vi "CalcTheta.vi"() -> (3 "ThetaValues":dbl[](array[numeric]))   [LabVIEW 2018]
panel:
  # "Front of bot"
  # "L"
  # "W"
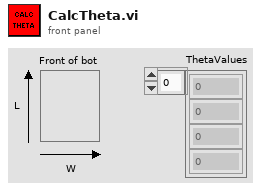
[diagram p1: front panel]
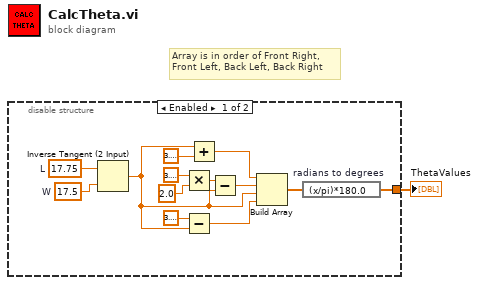
[diagram p0: block diagram]
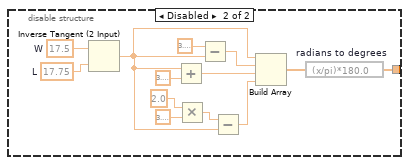
[diagram p2: hidden frame]
diagram:
  # "Array is in order of Front Right,\nFront Left, Back Left, Back Right"
  n1 = disable-structure shown="Enabled" {
    disable-tunnel: [w12 w22] -> w1
    frame Enabled {
      w11 = 17.75  # L
      w10 = 17.5  # W
      n2 = Inverse Tangent (2 Input)(1:w10, 2:w11) -> (0:w4:dbl)
      n3 = Multiply(x=3.141592653589793, y=2.0) -> (x*y=w6:dbl)
      n4 = Subtract(x=3.141592653589793, y=w4) -> (x-y=w3:dbl)
      n5 = Add(x=w4, y=3.141592653589793) -> (x+y=w2:dbl)
      n6 = Subtract(x=w6, y=w4) -> (x-y=w5:dbl)
      n7 = Build Array(w2, w5, w4, w3) -> (w9:dbl[])
      n8 = expression code="(x/pi)*180.0" "radians to degrees"(w9) -> (w12:dbl[])
    }
    frame Disabled {
      w20 = 17.5  # W
      w19 = 17.75  # L
      n9 = Inverse Tangent (2 Input)(1:w19, 2:w20) -> (0:w17:dbl)
      n10 = Add(x=w17, y=3.141592653589793) -> (x+y=w25:dbl)
      n11 = Multiply(x=2.0, y=3.141592653589793) -> (x*y=w16:dbl)
      n12 = Subtract(x=3.141592653589793, y=w17) -> (x-y=w21:dbl)
      n13 = Subtract(x=w16, y=w17) -> (x-y=w24:dbl)
      n14 = Build Array(w17, w21, w25, w24) -> (w23:dbl[])
      n15 = expression code="(x/pi)*180.0" "radians to degrees"(w23) -> (w22:dbl[])
    }
  }
  "ThetaValues" <- w1
